vi "setSuperKControls.vi"(2 "output cluster":T1, 6 "error in (no error)":errorcluster, 9 "COMport":string="COM6") -> (0 "error out":errorcluster)   [LabVIEW 2015]
uses:
  superKSDK/05_Labview Driver/Examples/To ByteArray ([U16]).vi
  superKSDK/05_Labview Driver/Examples/To ByteArray ([U32]).vi
panel:
  out "internalPulseFreqLimitHz":u32
  out "watchdogIntervalSec":u8
  out "burstPulses":u16
  out "internalPulseFreqHz":u16
  out "trigMode":u8
  out "displayBacklightPercent":u8
  out "trigLevelSetpointmV":u16
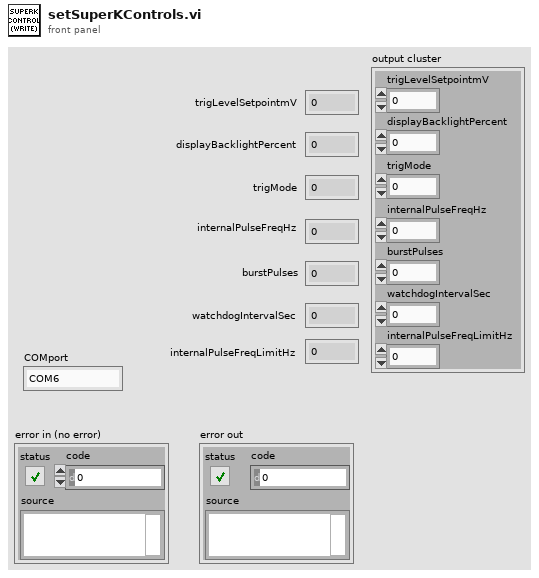
[diagram p1: front panel]
types:
  T1 = cluster{"trigLevelSetpointmV":u16, "displayBacklightPercent":u8, "trigMode":u8, "internalPulseFreqHz":u16, "burstPulses":u16, "watchdogIntervalSec":u8, "internalPulseFreqLimitHz":u32}
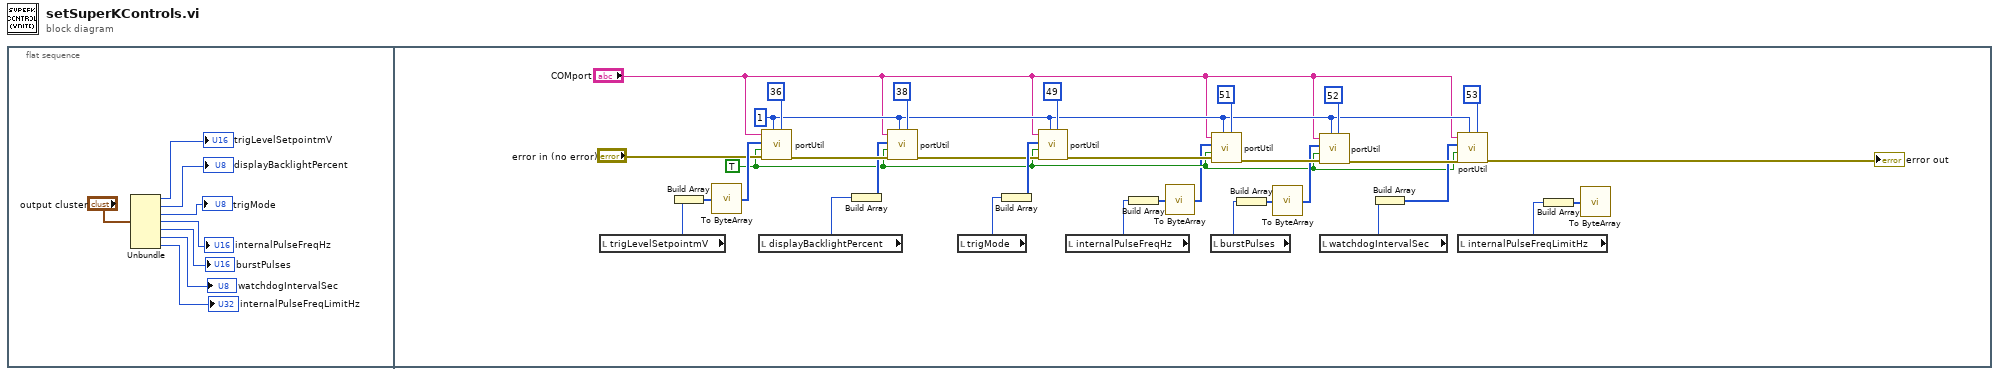
[diagram p0: block diagram]
diagram:
  n1 = flat-sequence {
    frame #0 {
      n2 = Unbundle("output cluster") -> ("trigLevelSetpointmV"=→"trigLevelSetpointmV":u16, "displayBacklightPercent"=→"displayBacklightPercent":u8, "trigMode"=→"trigMode":u8, "internalPulseFreqHz"=→"internalPulseFreqHz":u16, "burstPulses"=→"burstPulses":u16, "watchdogIntervalSec"=→"watchdogIntervalSec":u8, "internalPulseFreqLimitHz"=→"internalPulseFreqLimitHz":u32)
    }
    frame #1 {
      w10 = TRUE ("WriteNotRead")
      w25 = u8 1 ("Destination")
      n3 = local read "trigLevelSetpointmV"() -> (w18:u16)
      n4 = Build Array(w18) -> (w37:u16[])
      n5 = call-poly "To ByteArray.vi"("[U16]"=w37) -> ("PayloadByteArray"=w38:u8[])
      n6 = local read "displayBacklightPercent"() -> (w17:u8)
      n7 = call "portUtil.vi"("Register"=u8 36, "Destination"=w25, "error in (no error)"="error in (no error)", "WriteNotRead"=w10, "Array"=w38, "COMport"="COMport") -> ("error out"=w39:errorcluster)  [unwired: 3 in, 2 out]
      n8 = Build Array(w17) -> (w24:u8[])
      n9 = call "portUtil.vi"("Register"=u8 38, "Destination"=w25, "error in (no error)"=w39, "WriteNotRead"=w10, "Array"=w24, "COMport"="COMport") -> ("error out"=w21:errorcluster)  [unwired: 3 in, 2 out]
      n10 = local read "trigMode"() -> (w16:u8)
      n11 = Build Array(w16) -> (w23:u8[])
      n12 = call "portUtil.vi"("Register"=u8 49, "Destination"=w25, "error in (no error)"=w21, "WriteNotRead"=w10, "Array"=w23, "COMport"="COMport") -> ("error out"=w20:errorcluster)  [unwired: 3 in, 2 out]
      n13 = local read "internalPulseFreqHz"() -> (w15:u16)
      n14 = Build Array(w15) -> (w35:u16[])
      n15 = call-poly "To ByteArray.vi"("[U16]"=w35) -> ("PayloadByteArray"=w9:u8[])
      n16 = local read "burstPulses"() -> (w14:u16)
      n17 = call "portUtil.vi"("Register"=u8 51, "Destination"=w25, "error in (no error)"=w20, "WriteNotRead"=w10, "Array"=w9, "COMport"="COMport") -> ("error out"=w32:errorcluster)  [unwired: 3 in, 2 out]
      n18 = Build Array(w14) -> (w34:u16[])
      n19 = call-poly "To ByteArray.vi"("[U16]"=w34) -> ("PayloadByteArray"=w30:u8[])
      n20 = call "portUtil.vi"("Register"=u8 52, "Destination"=w25, "error in (no error)"=w32, "WriteNotRead"=w10, "Array"=w30, "COMport"="COMport") -> ("error out"=w31:errorcluster)  [unwired: 3 in, 2 out]
      n21 = local read "watchdogIntervalSec"() -> (w13:u8)
      n22 = Build Array(w13) -> (w22:u8[])
      n23 = call "portUtil.vi"("Register"=u8 53, "Destination"=w25, "error in (no error)"=w31, "WriteNotRead"=w10, "Array"=w22, "COMport"="COMport") -> ("error out"=→"error out":errorcluster)  [unwired: 3 in, 2 out]
      n24 = local read "internalPulseFreqLimitHz"() -> (w12:u32)
      n25 = Build Array(w12) -> (w33:u32[])
      n26 = call-poly "To ByteArray.vi"("[U32]"=w33) -> ()  [unwired: 1 out]
    }
  }
